vi "NI6008 DUT Switch.vi"(8 "error in (no error)":errorcluster, 10 "DUT No.":u8, 11 "Actor_NI6008 in":refnum<class "Actor_NI6008.lvclass">) -> (0 "error out":errorcluster, 3 "Actor_NI6008 out":refnum<class "Actor_NI6008.lvclass">)   [LabVIEW 2020, in "Actor_NI6008.lvlib" / "Actor_NI6008.lvclass"]
uses:
  Actor_NI6008.lvclass
  C:/Program Files/National Instruments/LabVIEW 2020/vi.lib/ActorFramework/Actor/Actor.lvclass
  <vilib>/ActorFramework/Actor/Actor.lvclass/Actor.ctl
  Actor_NI6008.lvclass/Actor_NI6008.ctl
  I_NI6008 Messages/NI6008 Status Report Msg/NI6008 Status Report Msg.lvclass/NI6008 Status Report Msg.ctl
  <vilib>/ActorFramework/Message Enqueuer/Message Enqueuer.lvclass/Message Enqueuer.ctl
  <vilib>/DAQmx/write.llb/DAQmx Write (Digital 1D Bool NChan 1Samp 1Line).vi
  <vilib>/ActorFramework/Message Enqueuer/Enqueue.vi
  I_NI6008 Messages/NI6008 Status Report Msg/NI6008 Status Report Msg.lvclass
  C:/Program Files/National Instruments/LabVIEW 2020/vi.lib/ActorFramework/Message/Message.lvclass
  <vilib>/DAQmx/miscellaneous.llb/DAQmx Fill In Error Info.vi
  <vilib>/ActorFramework/Message Priority Queue/Priority Enqueue.vi
  <vilib>/ActorFramework/Actor/Actor.lvclass
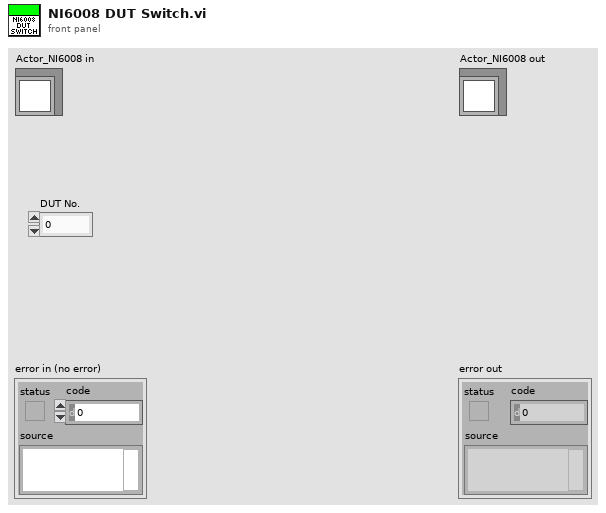
[diagram p1: front panel]
types:
  T1 = cluster{"Msg":string, "DO":bool[], "AI":dbl, "NI6008 Error":errorcluster}
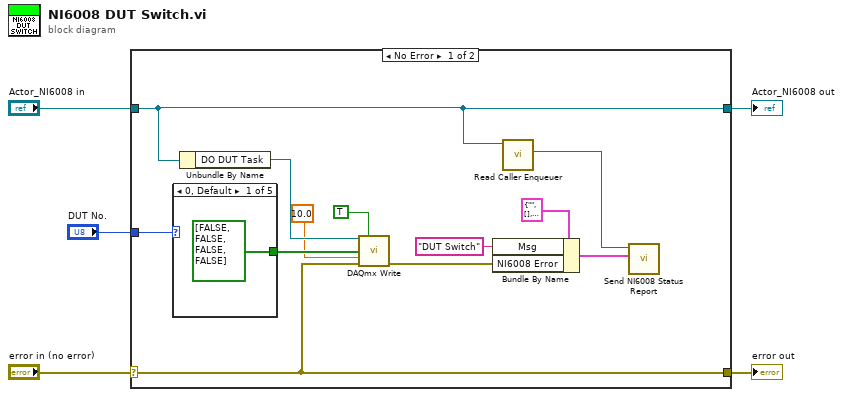
[diagram p0: block diagram]
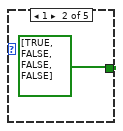
[diagram p2: hidden frame]
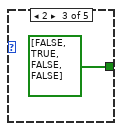
[diagram p3: hidden frame]
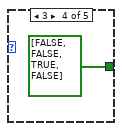
[diagram p4: hidden frame]
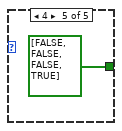
[diagram p5: hidden frame]
diagram:
  n1 = case shown="No Error" "error in (no error)" {
    selector: "error in (no error)" -> [w8 w24]
    tunnel: [w8 w24] -> w4
    tunnel: [w7 w23] -> w2
    tunnel: "Actor_NI6008 in" -> [w7 w23]
    tunnel: "DUT No." -> [w17 _]
    frame No Error {
      n2 = case shown="0, Default" w17 {
        tunnel: [bool[] [FALSE, FALSE, FALSE, FALSE] bool[] [TRUE, FALSE, FALSE, FALSE] bool[] [FALSE, TRUE, FALSE, FALSE] bool[] [FALSE, FALSE, TRUE, FALSE] bool[] [FALSE, FALSE, FALSE, TRUE]] -> w16
        frame 0, Default {
        }
        frame 1 {
        }
        frame 2 {
        }
        frame 3 {
        }
        frame 4 {
        }
      }
      n3 = Unbundle By Name(w7) -> ("DO DUT Task"=w15:refnum<k21>)
      n4 = call-poly <vilib>:"DAQmx Write.vi"("task/channels in"=w15, "auto start"=TRUE, "data"=w16, "timeout"=10.0, "error in"=w8) -> ("error out"=w10:errorcluster)  [unwired: 8 in, 2 out]
      n5 = Bundle By Name(cluster=T1 {"Msg"="", "DO"=[], "AI"=0.0, "NI6008 Error"={"status"=FALSE, "code"=0, "source"=""}} ("Data"), "Msg"="DUT Switch", "NI6008 Error"=w10) -> (w9:T1)
      n6 = call <vilib>:"Read Caller Enqueuer.vi"("Actor"=w7) -> ("Caller Enqueuer"=w6:refnum<class "Message Enqueuer.lvclass">)  [unwired: 10 in]
      n7 = call "Send NI6008 Status Report.vi"("Data"=w9, "Message Enqueuer"=w6) -> ()  [unwired: 8 in, 2 out]
    }
    frame Error {
    }
  }
  "error out" <- w4
  "Actor_NI6008 out" <- w2
